vi "Write Sequence.vi"(8 "error in (no error)":errorcluster, 10 "Sequence":bool, 11 "Variable in":refnum<class "Variable.lvclass">) -> (0 "error out":errorcluster, 3 "Variable out":refnum<class "Variable.lvclass">)   [LabVIEW 2013, in "Variable.lvclass"]
uses:
  Variable.lvclass
  Variable.lvclass/Variable.ctl
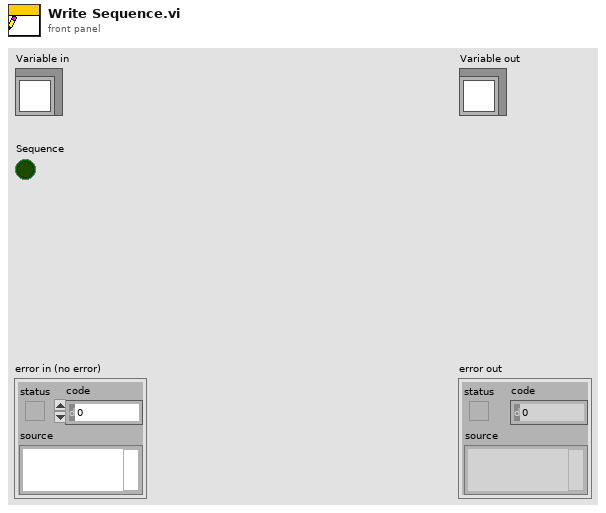
[diagram p1: front panel]
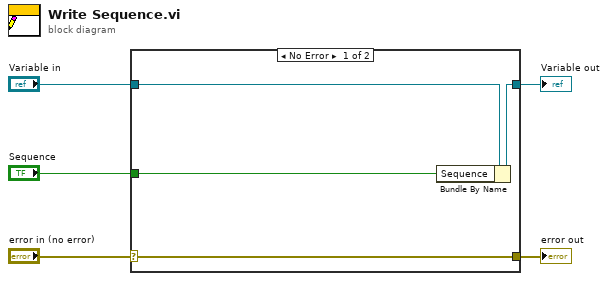
[diagram p0: block diagram]
diagram:
  n1 = case shown="No Error" "error in (no error)" {
    selector: "error in (no error)" -> [w9 w10]
    tunnel: [w9 w10] -> w4
    tunnel: [w7 w11] -> w2
    tunnel: "Variable in" -> [w8 w11]
    tunnel: "Sequence" -> [w6 _]
    frame No Error {
      n2 = Bundle By Name(cluster=w8, "Sequence"=w6) -> (w7:refnum<class "Variable.lvclass">)
    }
    frame Error {
    }
  }
  "error out" <- w4
  "Variable out" <- w2
